vi "New.vi"(8 "error in (no error)":errorcluster, 11 "Server Path":path) -> (0 "error out":errorcluster, 3 "PyServer out":refnum<class "PyServer.lvclass">)   [LabVIEW 2025, in "Tools.lvlib" / "PyServer.lvclass"]
uses:
  PyServer.lvclass
  PyServer.lvclass/PyServer.ctl
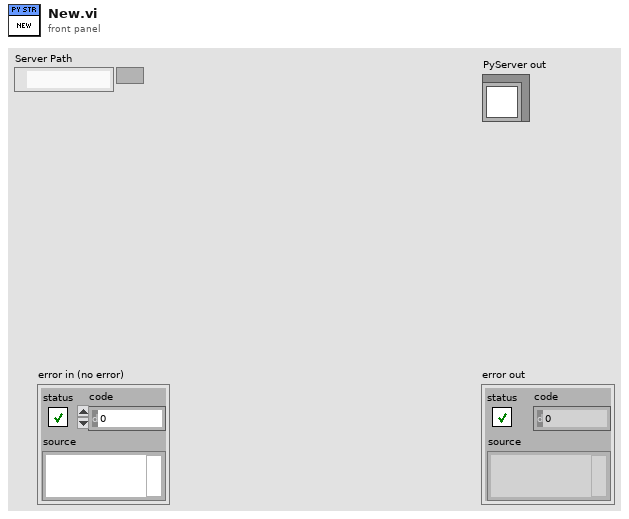
[diagram p1: front panel]
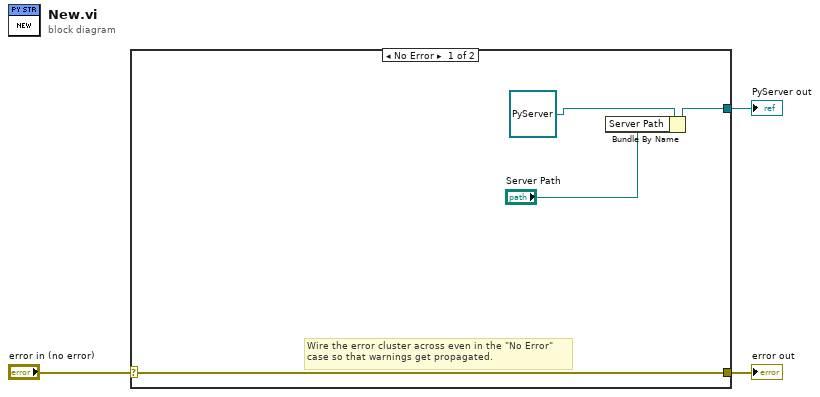
[diagram p0: block diagram]
diagram:
  n1 = case shown="No Error" "error in (no error)" {
    selector: "error in (no error)" -> [w7 w8]
    tunnel: [w7 w8] -> w2
    tunnel: [w5 _] -> w1
    frame No Error {
      # "Wire the error cluster across even in the \"No Error\"\ncase so that warnings get propagated."
      n2 = Bundle By Name(cluster=refnum<class "PyServer.lvclass"> refnum ("PyServer out"), "Server Path"="Server Path") -> (w5:refnum<class "PyServer.lvclass">)
    }
    frame Error {
    }
  }
  "error out" <- w2
  "PyServer out" <- w1
